vi "VISAwrite&Read.vi"() -> ()   [LabVIEW 2021]
panel:
  out "read buffer":string
  in  "write buffer":string
  in  "VISA resource name":refnum<visa-resource-name>
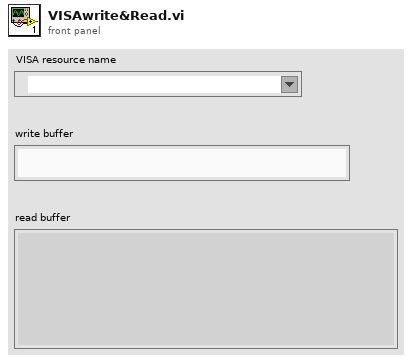
[diagram p1: front panel]
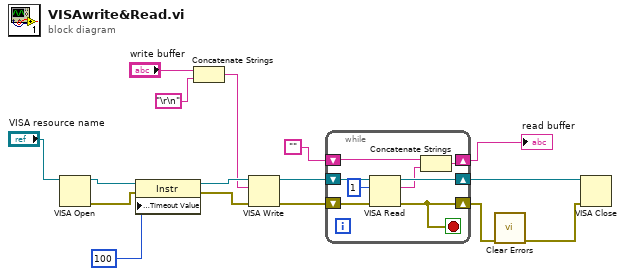
[diagram p0: block diagram]
diagram:
  n1 = VISA Open(VISA resource name="VISA resource name") -> (VISA resource name=w7:refnum<visa-resource-name>, error out=w6:errorcluster)  [unwired: 4 in]
  n2 = property class="Instr"(reference=w7, error in=w6, "General Settings:Timeout Value"=u32 100) -> (reference out=w5:refnum<visa-resource-name>, error out=w4:errorcluster)
  n3 = Concatenate Strings("write buffer", "\r\n") -> (w2:string)
  n4 = VISA Write(VISA resource name=w5, write buffer=w2, error in (no error)=w4) -> (VISA resource name out=w16:refnum<visa-resource-name>, error out=w15:errorcluster)  [unwired: 1 out]
  n5 = while {
    shift-right: [w22] -> w14
    shift-left: w16 -> [w24]
    shift-right: [w20] -> w13
    shift-left: w15 -> [w23]
    shift-right: [w18] -> w9
    shift-left: "" -> [w17]
    stop <- w20 stop-if-true
    n6 = VISA Read(VISA resource name=w24, byte count=u32 1, error in (no error)=w23) -> (VISA resource name out=w22:refnum<visa-resource-name>, read buffer=w19:string, error out=w20:errorcluster)  [unwired: 1 out]
    n7 = Concatenate Strings(w17, w19) -> (w18:string)
  }
  "read buffer" <- w9
  n8 = call <vilib>:"Clear Errors.vi"("error in (no error)"=w13) -> ("error out"=w3:errorcluster)  [unwired: 5 in, 1 out]
  n9 = VISA Close(VISA resource name=w14, error in (no error)=w3) -> ()  [unwired: 1 out]
